vi "RGB Color To Hue HSB.vi"(10 "Color":u32(colorbox)) -> (2 "HSB":T1)   [LabVIEW 2020, in "LMH-Hue.lvlib"]
doc: "This VI converts an RGB color into an HSB color calibrated for use with the Hue Lights (not quite standard HSB, two scaling constants are different)"
uses:
  LMH-Hue.lvlib
  Type Defs/HSB.ctl
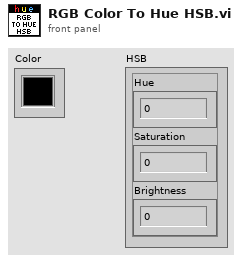
[diagram p1: front panel]
types:
  T1 = typedef "LMH-Hue.lvlib/HSB.ctl" = cluster{"Hue":u16, "Saturation":u8, "Brightness":u8}
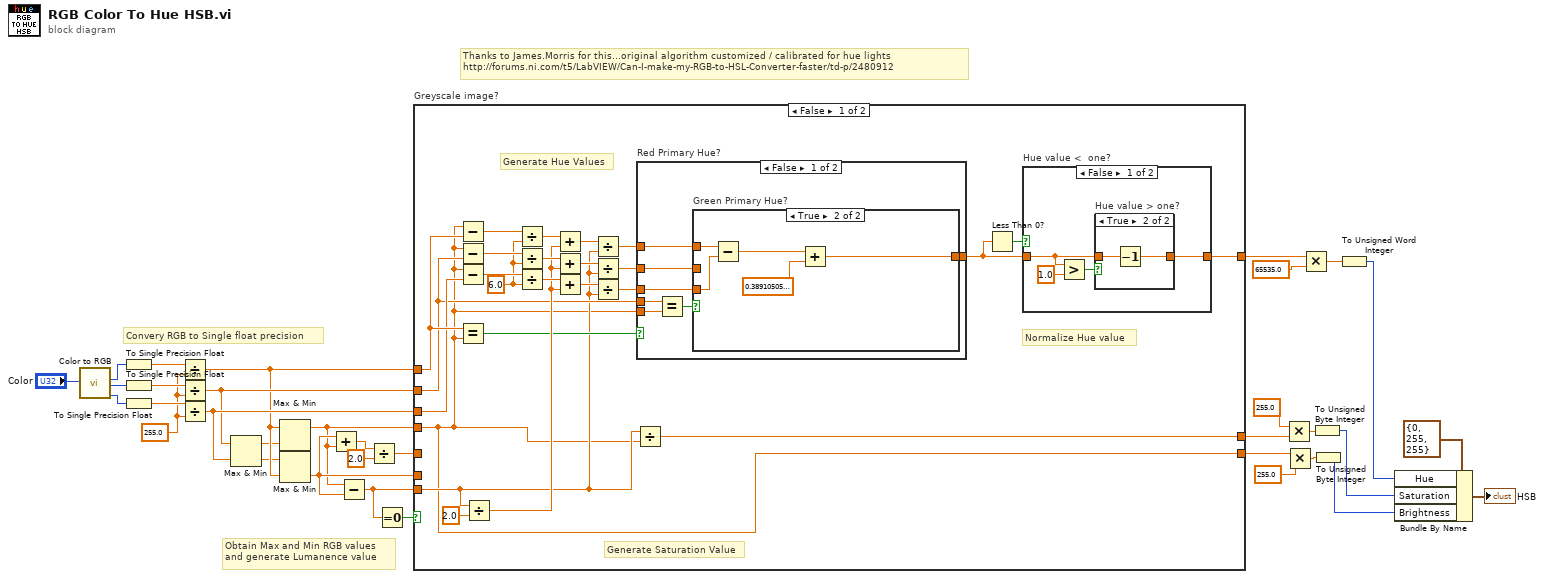
[diagram p0: block diagram]
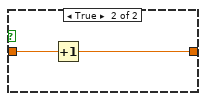
[diagram p3: hidden frame]
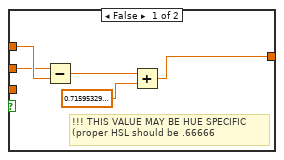
[diagram p4: hidden frame]
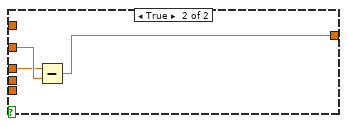
[diagram p5: hidden frame]
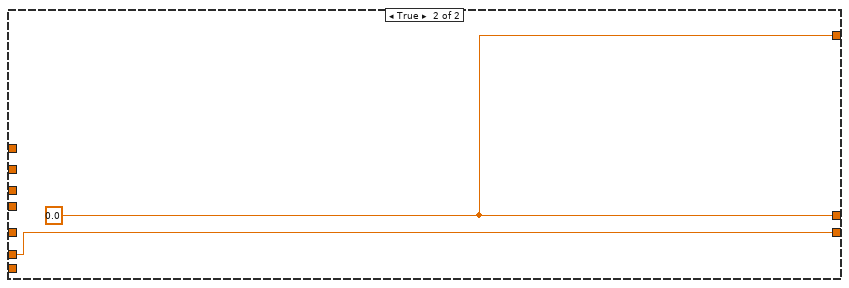
[diagram p6: hidden frame]
diagram:
  w11 = sgl 255.0 ("y")
  # "Thanks to James.Morris for this...original algorithm customized / calibrated for hue lights\nhttp://forums.ni.com/t5/LabVIEW/Can-I-make-my-RGB-to-HSL-Converter-faster/td-p/2480912"
  # "Convery RGB to Single float precision"
  # "Obtain Max and Min RGB values\nand generate Lumanence value"
  n1 = call <vilib>:"Color to RGB.vi"("Color"="Color") -> ("R"=w20:u8, "G"=w21:u8, "B"=w22:u8)  [unwired: 1 out]
  n2 = To Single Precision Float(number=w20) -> (single precision float=w17:sgl)
  n3 = To Single Precision Float(number=w21) -> (single precision float=w16:sgl)
  n4 = To Single Precision Float(number=w22) -> (single precision float=w15:sgl)
  n5 = Divide(x=w17, y=w11) -> (x/y=w8:sgl)
  n6 = Divide(x=w16, y=w11) -> (x/y=w9:sgl)
  n7 = Divide(x=w15, y=w11) -> (x/y=w10:sgl)
  n8 = Max & Min(x=w9, y=w10) -> (max(x,y)=w2:sgl, min(x,y)=w3:sgl)
  n9 = Max & Min(x=w8, y=w2) -> (max(x,y)=w5:sgl)  [unwired: 1 out]
  n10 = Max & Min(x=w3, y=w8) -> (min(x,y)=w6:sgl)  [unwired: 1 out]
  n11 = Add(x=w6, y=w5) -> (x+y=w14:sgl)
  n12 = Subtract(x=w5, y=w6) -> (x-y=w12:sgl)
  n13 = Divide(x=w14, y=sgl 2.0) -> (x/y=w7:sgl)
  n14 = Equal To 0?(x=w12) -> (x = 0?=w13:bool)
  n15 = case "Greyscale image?" shown="False" w13 {
    tunnel: w5 -> [w35 _]
    tunnel: w6 -> [_ w89]
    tunnel: w7 -> [_ _]
    tunnel: w10 -> [w42 _]
    tunnel: w9 -> [w41 _]
    tunnel: w8 -> [w43 _]
    tunnel: w12 -> [w37 _]
    tunnel: [w38 w90] -> w23
    tunnel: [w36 w90] -> w29
    tunnel: [w35 w89] -> w30
    frame False {
      w48 = sgl 6.0 ("y")
      # "Normalize Hue value"
      # "Generate Hue Values"
      # "Generate Saturation Value"
      n16 = Subtract(x=w35, y=w43) -> (x-y=w59:sgl)
      n17 = Subtract(x=w35, y=w41) -> (x-y=w58:sgl)
      n18 = Subtract(x=w35, y=w42) -> (x-y=w57:sgl)
      n19 = Equal?(x=w43, y=w35) -> (x = y?=w47:bool)
      n20 = Divide(x=w37, y=sgl 2.0) -> (x/y=w49:sgl)
      n21 = Divide(x=w59, y=w48) -> (x/y=w55:sgl)
      n22 = Divide(x=w58, y=w48) -> (x/y=w54:sgl)
      n23 = Divide(x=w57, y=w48) -> (x/y=w53:sgl)
      n24 = Add(x=w55, y=w49) -> (x+y=w50:sgl)
      n25 = Add(x=w54, y=w49) -> (x+y=w51:sgl)
      n26 = Add(x=w53, y=w49) -> (x+y=w52:sgl)
      n27 = Divide(x=w50, y=w37) -> (x/y=w44:sgl)
      n28 = Divide(x=w51, y=w37) -> (x/y=w45:sgl)
      n29 = Divide(x=w52, y=w37) -> (x/y=w46:sgl)
      n30 = Divide(x=w37, y=w35) -> (x/y=w36:sgl)
      n31 = case "Red Primary Hue?" shown="False" w47 {
        tunnel: w46 -> [w70 w87]
        tunnel: w45 -> [w71 w88]
        tunnel: w44 -> [w72 _]
        tunnel: w41 -> [w75 _]
        tunnel: w35 -> [w74 _]
        tunnel: [w69 w86] -> w39
        frame False {
          n32 = Equal?(x=w75, y=w74) -> (x = y?=w73:bool)
          n33 = case "Green Primary Hue?" shown="True" w73 {
            tunnel: w72 -> [w80 w85]
            tunnel: w71 -> [w76 _]
            tunnel: w70 -> [_ w84]
            tunnel: [w77 w81] -> w69
            frame False {
              # "!!! THIS VALUE MAY BE HUE SPECIFIC\n(proper HSL should be .66666"
              n34 = Subtract(x=w76, y=w80) -> (x-y=w79:sgl)
              n35 = Add(x=w79, y=sgl 0.7159533) -> (x+y=w77:sgl)
            }
            frame True {
              n36 = Subtract(x=w85, y=w84) -> (x-y=w83:sgl)
              n37 = Add(x=w83, y=sgl 0.38910505) -> (x+y=w81:sgl)
            }
          }
        }
        frame True {
          n38 = Subtract(x=w87, y=w88) -> (x-y=w86:sgl)
        }
      }
      n39 = Less Than 0?(x=w39) -> (x < 0?=w40:bool)
      n40 = case "Hue value <  one?" shown="False" w40 {
        tunnel: w39 -> [w60 w68]
        tunnel: [w61 w67] -> w38
        frame False {
          n41 = Greater?(x=w60, y=sgl 1.0) -> (0:w62:bool)
          n42 = case "Hue value > one?" shown="True" w62 {
            tunnel: w60 -> [w64 w66]
            tunnel: [w64 w65] -> w61
            frame False {
            }
            frame True {
              n43 = Decrement(x=w66) -> (x-1=w65:sgl)
            }
          }
        }
        frame True {
          n44 = Increment(x=w68) -> (x+1=w67:sgl)
        }
      }
    }
    frame True {
      w90 = sgl 0.0
    }
  }
  n45 = Multiply(x=sgl 255.0 ("y"), y=w29) -> (x*y=w31:sgl)
  n46 = Multiply(x=w30, y=sgl 255.0) -> (x*y=w33:sgl)
  n47 = Multiply(x=w23, y=sgl 65535.0) -> (x*y=w25:sgl)
  n48 = To Unsigned Byte Integer(number=w31) -> (unsigned 8bit integer=w32:u8)
  n49 = To Unsigned Byte Integer(number=w33) -> (unsigned 8bit integer=w34:u8)
  n50 = To Unsigned Word Integer(number=w25) -> (unsigned 16bit integer=w26:u16)
  n51 = Bundle By Name(cluster=T1 {"Hue"=0, "Saturation"=255, "Brightness"=255} ("HSB"), "Hue"=w26, "Saturation"=w32, "Brightness"=w34) -> (→"HSB":T1)
